vi "Read Asssertion Parameters 2.vi"(7 "Section":string, 8 "error in (no error)":errorcluster, 10 "Macro Step":T1, 11 "refnum":T5) -> (0 "error out":errorcluster, 2 "Macro Step out":T1={"Type"=enum."Mouse Move", "X"=0, "Y"=0, "Delay"=0, "Key"=65, "Repeat"=0, "RClick?"=FALSE, "App/Window Name"="", "Notes"="", "Assertion Type"=enum."Control Position", "Control Name"="", "Disabled"=enum."Enabled", "Visible"=enum."Visible", "Left"=0, "Top"=0, "Width"=0, "Height"=0, "Expected Image"={"image type"=0, "image depth"=0, "image"=[], "mask"=[], "colors"=[], "Rectangle"={"left"=0, "top"=0, "right"=0, "bottom"=0}}}, 3 "refnum out":T5)   [LabVIEW 2020, in "MacroAssert.lvlib"]
doc: "Reads the list of steps from macro config file defined by <B>refnum</B>."
uses:
  MacroAssert.lvlib
  <vilib>/ErrorRing/Error Ring.xnode
  <vilib>/Utility/config.llb/NI_LVConfig.lvlib
  <vilib>/Utility/config.llb/Read Key (I32).vi
  <vilib>/picture/picture.llb/imagedata.ctl
  <vilib>/Utility/error.llb/Error Cluster From Error Code.vi
  <vilib>/Utility/config.llb/Read Key (String).vi
  <vilib>/Utility/config.llb/Config Data RefNum.ctl
  CTLs/Step Type V3.ctl
  CTLs/Step V3.ctl
  CTLs/Assertion Type.ctl
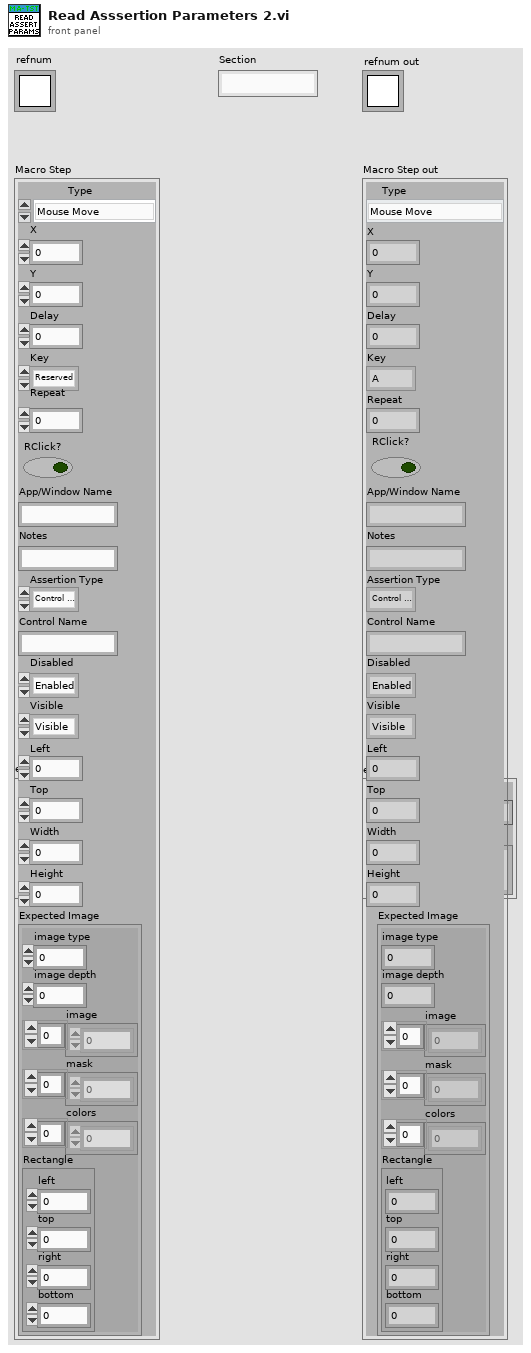
[diagram p1: front panel]
types:
  T1 = typedef "MacroAssert.lvlib/Step V3.ctl" = cluster{"Type":T2, "X":i32, "Y":i32, "Delay":i32, "Key":u8, "Repeat":i32, "RClick?":bool, "App/Window Name":string, "Notes":string, "Assertion Type":T3, "Control Name":string, "Disabled":enum8{"Enabled", "Disabled", "Disabled and Grayed Out"}, "Visible":enum16{"Visible", "Not Visible"}, "Left":i16, "Top":i16, "Width":i16, "Height":i16, "Expected Image":T4}
  T2 = typedef "MacroAssert.lvlib/Step Type V3.ctl" = enum16{"Mouse Move", "Mouse Click", "Key Press", "Wait", "Mouse Down", "Mouse Up", "Key Down", "Key Up", "Test Assertion", "Run Application", "Maximize Window", "Restore Window", "Minimize Window", "Close Window", "Bring Window to Front", "Send Window to Back"}
  T3 = typedef "MacroAssert.lvlib/Assertion Type.ctl" = enum16{"Control Position", "Control Visible", "Control Disabled", "Control Image"}
  T4 = typedef "imagedata.ctl" = cluster{"image type":i32, "image depth":i32, "image":u8[], "mask":u8[], "colors":u32[], "Rectangle":cluster{"left":i16, "top":i16, "right":i16, "bottom":i16}}
  T5 = typedef "NI_LVConfig.lvlib/Config Data RefNum.ctl" = refnum<k1>
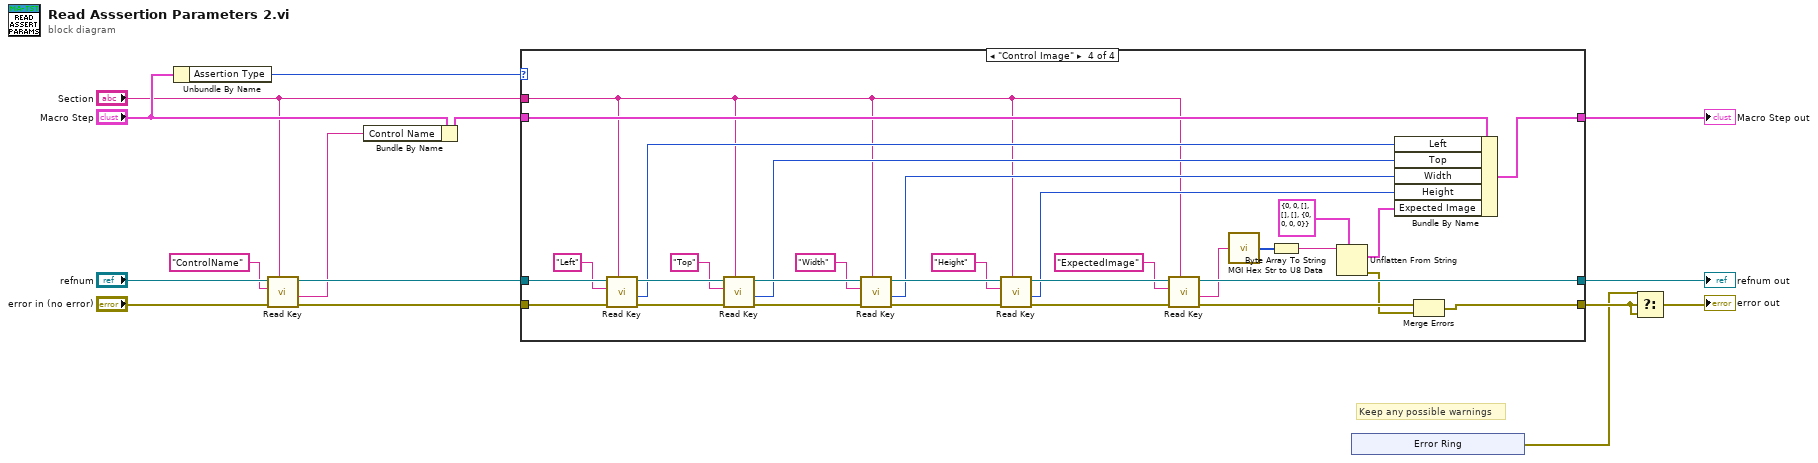
[diagram p0: block diagram]
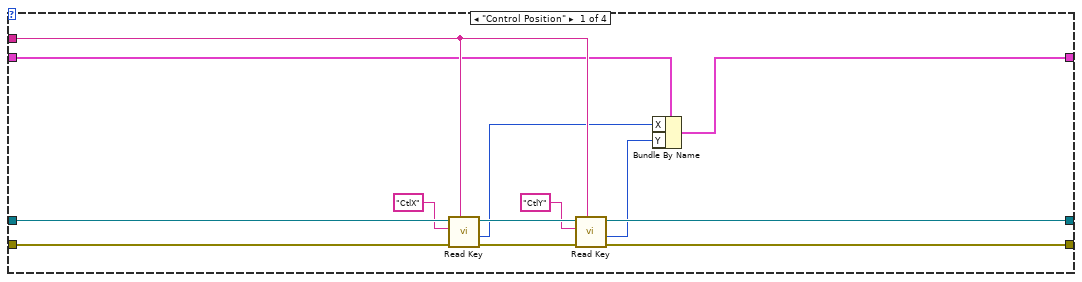
[diagram p2: hidden frame]
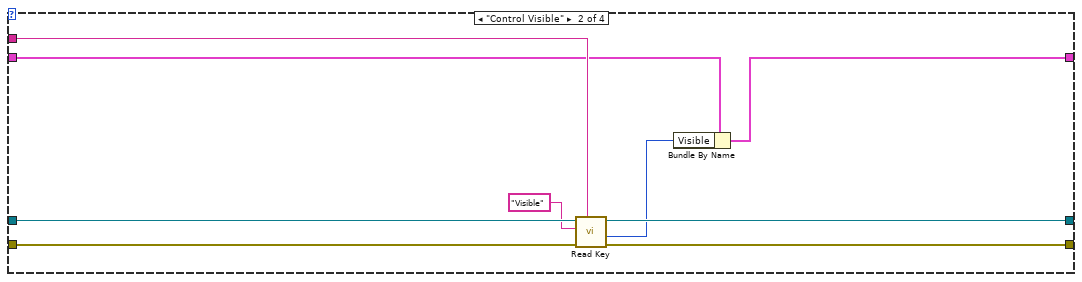
[diagram p3: hidden frame]
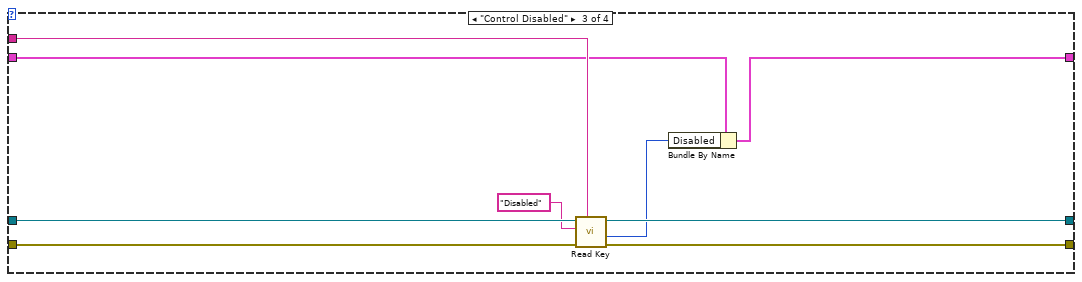
[diagram p4: hidden frame]
diagram:
  # "Keep any possible warnings"
  n1 = Unbundle By Name("Macro Step") -> ("Assertion Type"=w9:T3)
  n2 = call-poly <vilib>:"Read Key.vi"("section"="Section", "error in (no error)"="error in (no error)", "key"="ControlName", "refnum"="refnum") -> ("error out"=w7:errorcluster, "value"=w1:string, "refnum out"=w5:T5)  [unwired: 4 in, 1 out]
  n3 = Bundle By Name(cluster="Macro Step", "Control Name"=w1) -> (w2:T1)
  n4 = case shown="\"Control Image\"" w9 {
    tunnel: w7 -> [w28 w37 w46 w48]
    tunnel: w5 -> [w24 w35 w44 w77]
    tunnel: "Section" -> [w21 w33 w42 w47]
    tunnel: [w26 w36 w45 w62] -> w15
    tunnel: [w20 w32 w41 w70] -> w11
    tunnel: [w17 w30 w39 w69] -> w10
    tunnel: w2 -> [w16 w29 w38 w68]
    frame "Control Position" {
      n5 = call-poly <vilib>:"Read Key.vi"("section"=w21, "error in (no error)"=w28, "key"="CtlX", "refnum"=w24) -> ("error out"=w27:errorcluster, "value"=w19:i32, "refnum out"=w25:T5)  [unwired: 4 in, 1 out]
      n6 = call-poly <vilib>:"Read Key.vi"("section"=w21, "error in (no error)"=w27, "key"="CtlY", "refnum"=w25) -> ("error out"=w26:errorcluster, "value"=w18:i32, "refnum out"=w20:T5)  [unwired: 4 in, 1 out]
      n7 = Bundle By Name(cluster=w16, "X"=w19, "Y"=w18) -> (w17:T1)
    }
    frame "Control Visible" {
      n8 = call-poly <vilib>:"Read Key.vi"("section"=w33, "error in (no error)"=w37, "key"="Visible", "refnum"=w35) -> ("error out"=w36:errorcluster, "value"=w31:i32, "refnum out"=w32:T5)  [unwired: 4 in, 1 out]
      n9 = Bundle By Name(cluster=w29, "Visible"=w31) -> (w30:T1)
    }
    frame "Control Disabled" {
      n10 = call-poly <vilib>:"Read Key.vi"("section"=w42, "error in (no error)"=w46, "key"="Disabled", "refnum"=w44) -> ("error out"=w45:errorcluster, "value"=w40:i32, "refnum out"=w41:T5)  [unwired: 4 in, 1 out]
      n11 = Bundle By Name(cluster=w38, "Disabled"=w40) -> (w39:T1)
    }
    frame "Control Image" {
      n12 = call-poly <vilib>:"Read Key.vi"("section"=w47, "error in (no error)"=w48, "key"="Left", "refnum"=w77) -> ("error out"=w56:errorcluster, "value"=w52:i32, "refnum out"=w76:T5)  [unwired: 4 in, 1 out]
      n13 = call-poly <vilib>:"Read Key.vi"("section"=w47, "error in (no error)"=w56, "key"="Top", "refnum"=w76) -> ("error out"=w55:errorcluster, "value"=w51:i32, "refnum out"=w75:T5)  [unwired: 4 in, 1 out]
      n14 = call-poly <vilib>:"Read Key.vi"("section"=w47, "error in (no error)"=w55, "key"="Width", "refnum"=w75) -> ("error out"=w54:errorcluster, "value"=w50:i32, "refnum out"=w74:T5)  [unwired: 4 in, 1 out]
      n15 = call-poly <vilib>:"Read Key.vi"("section"=w47, "error in (no error)"=w54, "key"="Height", "refnum"=w74) -> ("error out"=w53:errorcluster, "value"=w49:i32, "refnum out"=w73:T5)  [unwired: 4 in, 1 out]
      n16 = call-poly <vilib>:"Read Key.vi"("section"=w47, "error in (no error)"=w53, "key"="ExpectedImage", "refnum"=w73) -> ("error out"=w72:errorcluster, "value"=w67:string, "refnum out"=w70:T5)  [unwired: 4 in, 1 out]
      n17 = call <userlib>:"MGI Hex Str to U8 Data.vi"("HEX String (0-9,A-F)"=w67) -> ("u8 Data[]"=w66:u8[])
      n18 = Byte Array To String(unsigned byte array=w66) -> (string=w65:string)
      n19 = Unflatten From String(type=T4 {"image type"=0, "image depth"=0, "image"=[], "mask"=[], "colors"=[], "Rectangle"={"left"=0, "top"=0, "right"=0, "bottom"=0}} ("Expected Image"), binary string=w65) -> (value=w63:T4, error out=w61:errorcluster)  [unwired: 3 in, 1 out]
      n20 = Bundle By Name(cluster=w68, "Left"=w52, "Top"=w51, "Width"=w50, "Height"=w49, "Expected Image"=w63) -> (w69:T1)
      n21 = Merge Errors(w72, w61) -> (w62:errorcluster)
    }
  }
  "refnum out" <- w11
  "Macro Step out" <- w10
  n22 = xnode "Error Ring"() -> ("error out"=w14:errorcluster)
  n23 = Select(t=w14, s=w15, f=w15) -> (s? t:f=→"error out":errorcluster)
